vi "Init Module.vi"(8 "error in (no error)":errorcluster, 11 "Cloneable Module Admin in":refnum<class "Delacor_lib_QMH_Cloneable Module Admin.lvclass">) -> (0 "error out":errorcluster, 2 "LGP5 Acquisition Request Events":T1, 3 "Cloneable Module Admin out":refnum<class "Delacor_lib_QMH_Cloneable Module Admin.lvclass">)   [LabVIEW 2018, in "LGP5 Acquisition.lvlib"]
doc: "Initialize the module by creating Broadcast Events, Request Events, and synchronization rendezvous. Also, since this is a cloneable module, add it to the cloneable registry and update the Module Admin class.\n_____\nBased on Delacor QMH Project Template 4.1.0.59."
uses:
  LGP5 Acquisition.lvlib
  <vilib>/Delacor/Delacor QMH/Libraries/Cloneable Module Admin_class/Delacor_lib_QMH_Cloneable Module Admin.lvclass
  C:/Program Files (x86)/National Instruments/LabVIEW 2018/vi.lib/Delacor/Delacor QMH/Libraries/Module Admin_class/Delacor_lib_QMH_Module Admin.lvclass
  Request Events--cluster.ctl
  Stop Argument--cluster.ctl
  Show Panel Argument--cluster.ctl
  Hide Panel Argument--cluster.ctl
  Show Diagram Argument--cluster.ctl
  Get Module Execution Status Argument--cluster.ctl
  Start Acquiring Argument--cluster.ctl
  Start Acquiring (Reply Payload)--cluster.ctl
  Stop Acquiring Argument--cluster.ctl
  Stop Acquiring (Reply Payload)--cluster.ctl
  Wake Up Helper Loop Argument--cluster.ctl
  <vilib>/Delacor/Delacor QMH/Libraries/Module Admin_class/Delacor_lib_QMH_Module Admin.lvclass/Delacor_lib_QMH_Module Admin.ctl
  <vilib>/Delacor/Delacor QMH/Libraries/Cloneable Module Admin_class/Delacor_lib_QMH_Cloneable Module Admin.lvclass/Delacor_lib_QMH_Cloneable Module Admin.ctl
  <vilib>/Delacor/Delacor QMH/Libraries/Module Admin_class/Delacor_lib_QMH_Get External Launch.vi
  <vilib>/Delacor/Delacor QMH/Libraries/Cloneable Module Admin_class/Delacor_lib_QMH_Get Module ID.vi
  <vilib>/Delacor/Delacor QMH/Libraries/Cloneable Module Admin_class/Delacor_lib_QMH_Set First.vi
  Clone Registration/Clone Registration.lvlib
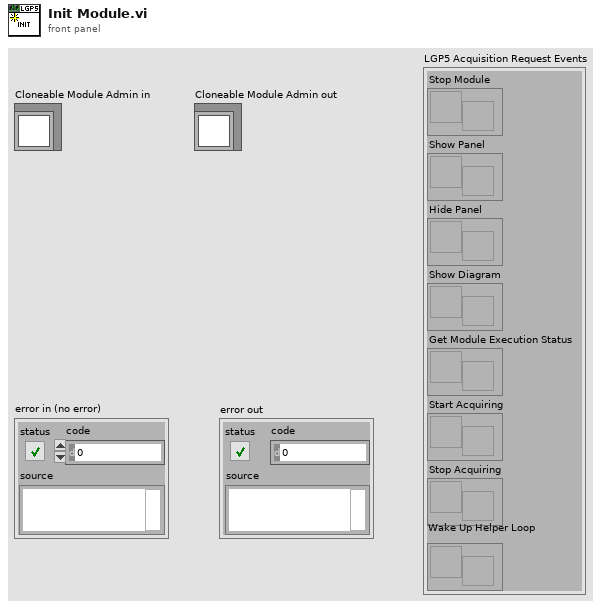
[diagram p1: front panel]
types:
  T1 = typedef "LGP5 Acquisition.lvlib/Request Events--cluster.ctl" = cluster{"Stop Module":refnum<user-event>, "Show Panel":refnum<user-event>, "Hide Panel":refnum<user-event>, "Show Diagram":refnum<user-event>, "Get Module Execution Status":refnum<user-event>, "Start Acquiring":refnum<user-event>, "Stop Acquiring":refnum<user-event>, "Wake Up Helper Loop":refnum<user-event>}
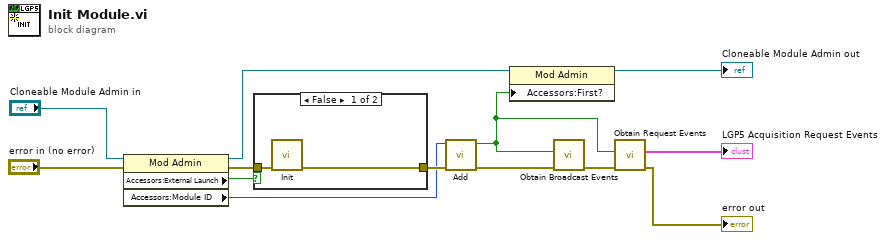
[diagram p0: block diagram]
diagram:
  n1 = property class="Mod Admin"(reference="Cloneable Module Admin in", error in="error in (no error)") -> (reference out=w7:refnum<class "Delacor_lib_QMH_Cloneable Module Admin.lvclass">, error out=w2:errorcluster, "Accessors:External Launch"=w6:bool, "Accessors:Module ID"=w1:i32)
  n2 = case "External Launch?" shown="False" w6 {
    tunnel: [w15 w16] -> w12
    tunnel: w2 -> [w14 w16]
    frame False {
      n3 = call "Init.vi"("error in (no error)"=w14) -> ("error out"=w15:errorcluster)  [unwired: 7 in, 3 out]
    }
    frame True {
      # "Init of Clone's registration\nhappened at Start Module.vi"
    }
  }
  n4 = call "Add.vi"("error in (no error)"=w12, "Module ID"=w1) -> ("error out"=w13:errorcluster, "First?"=w8:bool)  [unwired: 7 in, 1 out]
  n5 = property class="Mod Admin"(reference=w7, "Accessors:First?"=w8) -> (reference out=→"Cloneable Module Admin out":refnum<class "Delacor_lib_QMH_Cloneable Module Admin.lvclass">)  [unwired: 1 in, 1 out]
  n6 = call "Obtain Broadcast Events.vi"("error in (no error)"=w13, "Create New? (F)"=w8) -> ("error out"=w11:errorcluster)  [unwired: 8 in, 1 out]
  n7 = call "Obtain Request Events.vi"("error in (no error)"=w11, "Create New? (F)"=w8) -> ("error out"=→"error out":errorcluster, "LGP5 Acquisition Request Events"=→"LGP5 Acquisition Request Events":T1)  [unwired: 8 in]
